vi "Close Module.vi"(8 "error in":errorcluster, 9 "Wait for stop?":bool, 11 "Module Admin in":refnum<class "Delacor_lib_QMH_Cloneable Module Admin.lvclass">) -> (0 "error out":errorcluster, 1 "External Launch":bool, 3 "Module Admin out":refnum<class "Delacor_lib_QMH_Cloneable Module Admin.lvclass">)   [LabVIEW 2020, in "My CloneableDQMH.lvlib"]
doc: "Destroy the Broadcast Events and Request Events (if this was the first instance). Reset flags stored in Module Admin class.\n_____\nBased on DQMH Project Template 6.0.0.91."
uses:
  My CloneableDQMH.lvlib
  <vilib>/Delacor/Delacor QMH/Libraries/Cloneable Module Admin_class/Delacor_lib_QMH_Cloneable Module Admin.lvclass
  C:/Program Files (x86)/National Instruments/LabVIEW 2020/vi.lib/Delacor/Delacor QMH/Libraries/Module Admin_class/Delacor_lib_QMH_Module Admin.lvclass
  <vilib>/Delacor/Delacor QMH/Libraries/Cloneable Module Admin_class/Delacor_lib_QMH_Cloneable Module Admin.lvclass/Delacor_lib_QMH_Cloneable Module Admin.ctl
  <vilib>/Delacor/Delacor QMH/Libraries/Module Admin_class/Delacor_lib_QMH_Module Admin.lvclass/Delacor_lib_QMH_Module Admin.ctl
  <vilib>/Delacor/Delacor QMH/Libraries/Cloneable Module Admin_class/Delacor_lib_QMH_Get First.vi
  <vilib>/Delacor/Delacor QMH/Libraries/Cloneable Module Admin_class/Delacor_lib_QMH_Get Module ID.vi
  <vilib>/Delacor/Delacor QMH/Libraries/Module Admin_class/Delacor_lib_QMH_Get External Launch.vi
  <vilib>/Delacor/Delacor QMH/Libraries/Cloneable Module Admin_class/Delacor_lib_QMH_Get Close Master Reference.vi
  Clone Registration/Clone Registration.lvlib
  VI Reference Management/VI Reference Management.lvlib
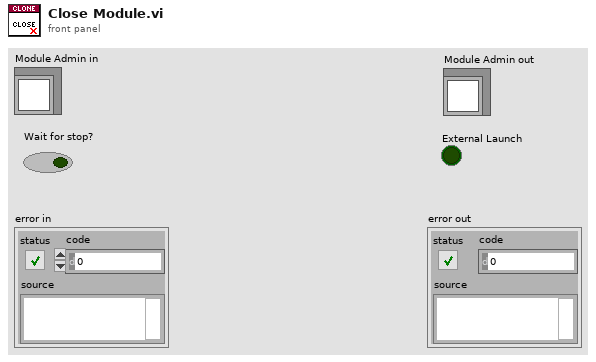
[diagram p1: front panel]
types:
  T1 = typedef "Semaphore RefNum" = refnum<k1>
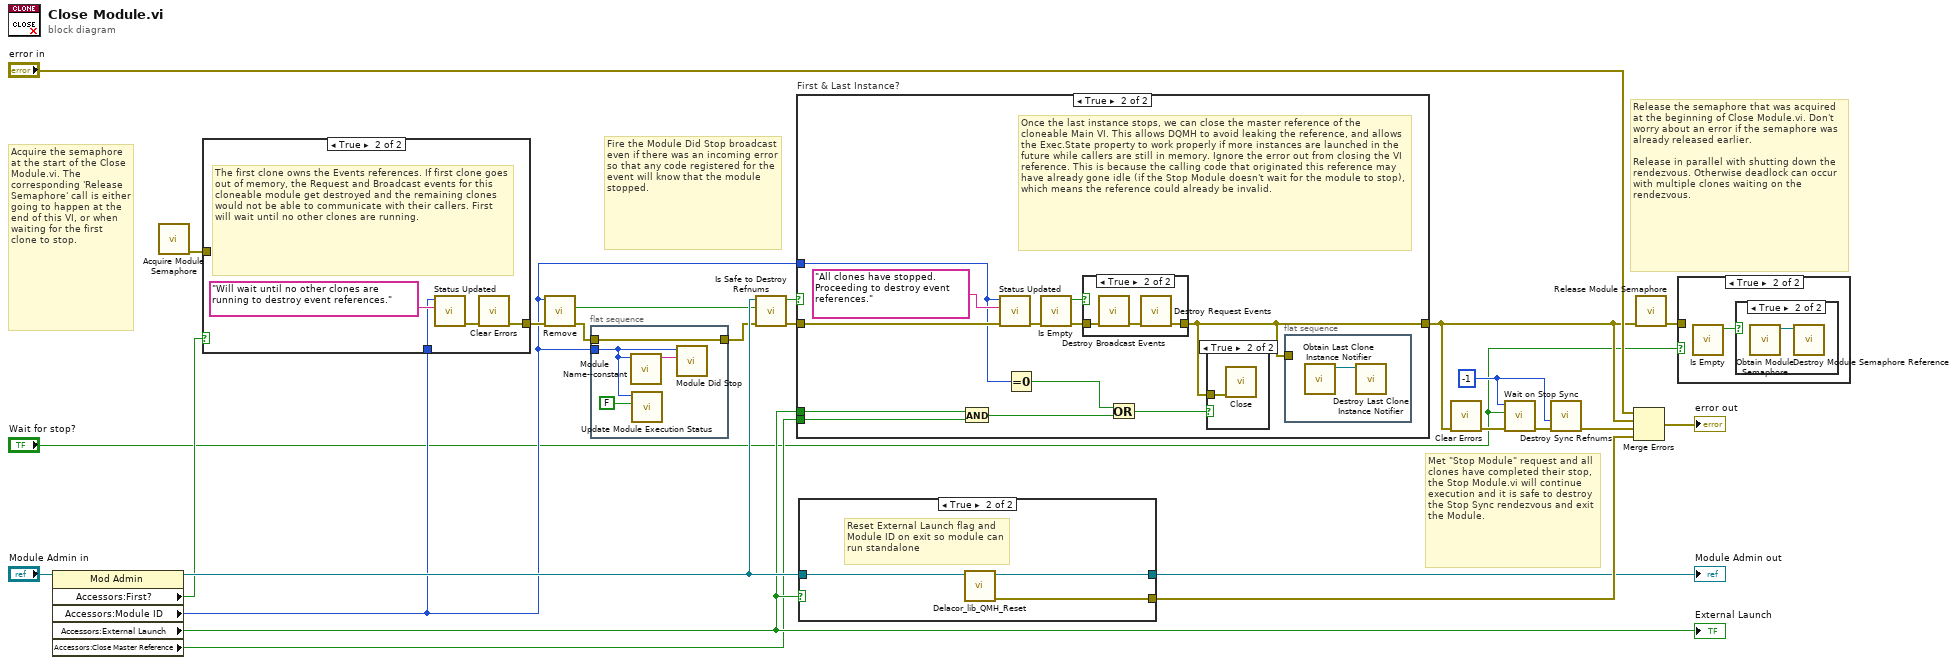
[diagram p0: block diagram]
diagram:
  w15 = -1 ("Module ID")
  # "Release the semaphore that was acquired at the beginning of Close Module.vi. Don't worry about an error if the semaphore was already released earlier.\n\nRelease in parallel with shutting down the rendezvous. Otherwise deadlock can occur with multiple clones waiting on the rendezvous."
  # "Acquire the semaphore at the start of the Close Module.vi. The corresponding 'Release Semaphore' call is either going to happen at the end of this VI, or when waiting for the first clone to stop."
  # "Fire the Module Did Stop broadcast even if there was an incoming error so that any code registered for the event will know that the module stopped."
  # "Met \"Stop Module\" request and all clones have completed their stop, the Stop Module.vi will continue execution and it is safe to destroy the Stop Sync rendezvous and exit the Module."
  n1 = property class="Mod Admin"(reference="Module Admin in") -> (reference out=w22:refnum<class "Delacor_lib_QMH_Cloneable Module Admin.lvclass">, "Accessors:First?"=w13:bool, "Accessors:Module ID"=w7:i32, "Accessors:External Launch"=w11:bool, "Accessors:Close Master Reference"=w6:bool)  [unwired: 1 in, 1 out]
  "External Launch" <- w11
  n2 = call "Acquire Module Semaphore.vi"() -> ("error out"=w5:errorcluster)  [unwired: 11 in]
  n3 = case shown="True" w13 {
    tunnel: w7 -> [_ w27]
    tunnel: [_ w25] -> w24
    tunnel: w5 -> [_ _]
    frame False {
    }
    frame True {
      # "The first clone owns the Events references. If first clone goes out of memory, the Request and Broadcast events for this cloneable module get destroyed and the remaining clones would not be able to communicate with their callers. First will wait until no other clones are running."
      n4 = call "Status Updated.vi"("Status"="Will wait until no other clones are running to destroy event references." ("format string"), "Module ID"=w27) -> ("error out"=w26:errorcluster)  [unwired: 9 in]
      n5 = call <vilib>:"Clear Errors.vi"("error in (no error)"=w26) -> ("error out"=w25:errorcluster)  [unwired: 5 in, 1 out]
    }
  }
  n6 = call "Remove.vi"("error in (no error)"=w24, "Module ID"=w7) -> ("error out"=w9:errorcluster, "empty"=w10:bool)  [unwired: 8 in]
  n7 = flat-sequence {
    tunnel: w9 -> [w32]
    tunnel: [w32] -> w8
    tunnel: w7 -> [w30]
    frame #0 {
      n8 = call "Module Name--constant.vi"("Module ID"=w30) -> ("Module Name"=w31:string)  [unwired: 10 in]
      n9 = call "Update Module Execution Status.vi"("Running?"=FALSE, "Module ID"=w30) -> ()  [unwired: 9 in, 1 out]
      n10 = call "Module Did Stop.vi"("Origin"=w31, "Module ID"=w30) -> ()  [unwired: 9 in, 1 out]
    }
  }
  n11 = call "Is Safe to Destroy Refnums.vi"("error in"=w8, "empty"=w10, "Module Admin"=w22) -> ("error out"=w19:errorcluster, "Destroy Broadcast & Request Event Refs?"=w20:bool)  [unwired: 7 in]
  n12 = case "First & Last Instance?" shown="True" w20 {
    tunnel: w19 -> [w33 w45]
    tunnel: [w33 w37] -> w3
    tunnel: w7 -> [_ w39]
    tunnel: w11 -> [_ w43]
    tunnel: w6 -> [_ w41]
    frame False {
    }
    frame True {
      # "Once the last instance stops, we can close the master reference of the cloneable Main VI. This allows DQMH to avoid leaking the reference, and allows the Exec.State property to work properly if more instances are launched in the future while callers are still in memory. Ignore the error out from closing the VI reference. This is because the calling code that originated this reference may have already gone idle (if the Stop Module doesn't wait for the module to stop), which means the reference could already be invalid."
      n13 = And(x=w43, y=w41) -> (x .and. y?=w42:bool)
      n14 = call "Status Updated.vi"("error in (no error)"=w45, "Status"="All clones have stopped. Proceeding to destroy event references.", "Module ID"=w39) -> ("error out"=w36:errorcluster)  [unwired: 8 in]
      n15 = Equal To 0?(x=w39) -> (x = 0?=w38:bool)
      n16 = call "Is Empty.vi"("error in (no error)"=w36) -> ("error out"=w35:errorcluster, "Empty?"=w34:bool)  [unwired: 9 in]
      n17 = case shown="True" w34 {
        tunnel: [w46 w48] -> w37
        tunnel: w35 -> [w46 w47]
        frame False {
        }
        frame True {
          n18 = call "Destroy Broadcast Events.vi"("error in (no error)"=w47) -> ("error out"=w49:errorcluster)  [unwired: 10 in]
          n19 = call "Destroy Request Events.vi"("error in (no error)"=w49) -> ("error out"=w48:errorcluster)  [unwired: 10 in]
        }
      }
      n20 = Or(x=w38, y=w42) -> (x .or. y?=w40:bool)
      n21 = case shown="True" w40 {
        tunnel: w37 -> [_ w51]
        frame False {
        }
        frame True {
          n22 = call "Close.vi"("error in (no error)"=w51) -> ()  [unwired: 10 in, 1 out]
        }
      }
      n23 = flat-sequence {
        tunnel: w37 -> [_]
        frame #0 {
          n24 = call "Obtain Last Clone Instance Notifier.vi"() -> ("Last Instance Notifier"=w50:refnum<notifier>)  [unwired: 10 in, 1 out]
          n25 = call "Destroy Last Clone Instance Notifier.vi"("Last Instance Notifier"=w50) -> ()  [unwired: 11 in]
        }
      }
    }
  }
  n26 = case shown="True" w11 {
    tunnel: w22 -> [w52 w55]
    tunnel: [w52 w54] -> w18
    tunnel: [_ w53] -> w23
    frame False {
    }
    frame True {
      # "Reset External Launch flag and Module ID on exit so module can run standalone"
      n27 = call-dynamic "Delacor_lib_QMH_Reset.vi"("Mod Admin in"=w55) -> ("error out"=w53:errorcluster, "Mod Admin out"=w54:refnum<class "Delacor_lib_QMH_Cloneable Module Admin.lvclass">)  [unwired: 9 in]
    }
  }
  "Module Admin out" <- w18
  n28 = call <vilib>:"Clear Errors.vi"("error in (no error)"=w3) -> ("error out"=w14:errorcluster)  [unwired: 5 in, 1 out]
  n29 = call "Wait on Stop Sync.vi"("error in (no error)"=w14, "Wait for Module to stop?"="Wait for stop?", "Module ID"=w15) -> ("error out"=w17:errorcluster)  [unwired: 8 in]
  n30 = call "Destroy Sync Refnums.vi"("error in (no error)"=w17, "Module ID"=w15) -> ("error out"=w16:errorcluster)  [unwired: 9 in]
  n31 = Merge Errors("error in", w3, w16, w23) -> (→"error out":errorcluster)
  n32 = call "Release Module Semaphore.vi"("error in"=w3) -> ("error out"=w2:errorcluster)  [unwired: 10 in]
  n33 = case shown="True" "Wait for stop?" {
    tunnel: w2 -> [_ _]
    frame False {
    }
    frame True {
      n34 = call "Is Empty.vi"() -> ("Empty?"=w56:bool)  [unwired: 10 in, 1 out]
      n35 = case shown="True" w56 {
        frame False {
        }
        frame True {
          n36 = call "Obtain Module Semaphore.vi"() -> ("semaphore"=w57:T1)  [unwired: 9 in, 2 out]
          n37 = call "Destroy Module Semaphore Reference.vi"("semaphore"=w57) -> ()  [unwired: 10 in, 1 out]
        }
      }
    }
  }
